vi "Coord window-Force apply setup.vi"   [LabVIEW 2017]
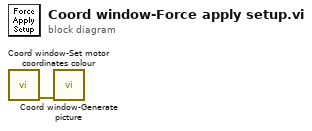
[diagram p0: block diagram]
diagram:
  n1 = call "Coord window-Set motor coordinates colour.vi"() -> ("error out"=w1:errorcluster)  [unwired: 11 in]
  n2 = call "Coord window-Generate picture.vi"("error in (no error)"=w1) -> ()  [unwired: 10 in, 1 out]
